vi "Operation Main.vi"(8 "error in (no error)":errorcluster, 11 "Parallel Operation Actor in":refnum<class "Parallel Operation Actor.lvclass">) -> (0 "error out":errorcluster, 3 "Parallel Operation Actor out":refnum<class "Parallel Operation Actor.lvclass">)   [LabVIEW 2024, in "Parallel Operation Actor.lvclass"]
uses:
  Parallel Operation Actor.lvclass
  Ancestor Class/Actor/System Actor/System Actor.lvclass
  Parallel Operation Actor.lvclass/Parallel Operation Actor.ctl
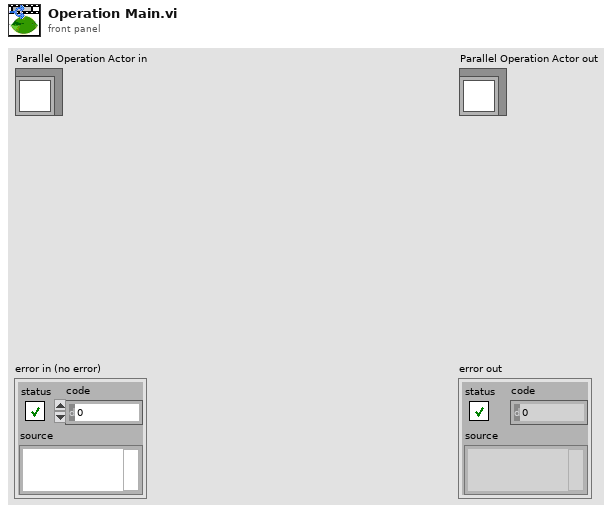
[diagram p1: front panel]
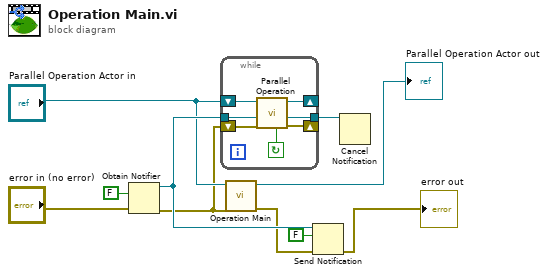
[diagram p0: block diagram]
diagram:
  n1 = Obtain Notifier(notification data type=FALSE, error in (no error)="error in (no error)") -> (notifier out=w9:refnum<notifier>, error out=w1:errorcluster)  [unwired: 2 in, 1 out]
  n2 = while {
    tunnel: w9 -> [w15]
    tunnel: [w14] -> w2
    shift-right: [w12] -> _
    shift-left: w1 -> [w13]
    shift-right: [w11] -> _
    shift-left: "Parallel Operation Actor in" -> [w17]
    stop <- w16 continue-if-true
    n3 = call-dynamic "Parallel Operation.vi"("error in (no error)"=w13, "Stop Notifier In"=w15, "Parallel Operation Actor in"=w17) -> ("error out"=w12:errorcluster, "Stop Notifier Out"=w14:refnum<notifier>, "Parallel Operation Actor out"=w11:refnum<class "Parallel Operation Actor.lvclass">, "Notifier Status"=w16:bool)  [unwired: 5 in]
  }
  n4 = call-parent "Operation Main.vi"("error in (no error)"=w1, "System Actor in"="Parallel Operation Actor in") -> ("error out"=w8:errorcluster, "System Actor out"=→"Parallel Operation Actor out":refnum<class "Parallel Operation Actor.lvclass">)  [unwired: 8 in]
  n5 = Send Notification(notification=FALSE, notifier=w9, error in (no error)=w8) -> (error out=→"error out":errorcluster)  [unwired: 1 out]
  n6 = Cancel Notification(0:w2) -> ()  [unwired: 1 in, 3 out]
